vi "One Button Dialog with Timeout.vi"(0 "message":string, 1 "Btn Timeout(-1 s)":i32=-1, 3 "T button name (\"OK\")":string="OK", 5 "Parent Wnd(Caller By Default)":refnum<vi>) -> (7 "true":bool)   [LabVIEW 2017]
doc: "Shows a one-button dialog carrying the message and the button name given, and closes it automatically after Btn Timeout(-1 s) seconds. A negative timeout disables the automatic close."
uses:
  a539abf7-d72e-4e1a-867b-c48a8ed28406.vi
panel:
  out "font":T1
  in  "btn":bool
  out "String":string
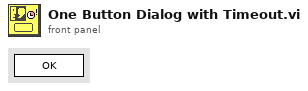
[diagram p1: front panel]
types:
  T1 = cluster{"Font Name:":string, "Size":i16, "Strikeout?":bool, "Italic?":bool, "Underline?":bool, "Outline?":bool, "Shadow?":bool, "Bold?":bool}
  T2 = typedef "LVFontTypeDef.ctl" = cluster{"Font Name":string, "Size":u16, "Bold":bool, "Italic":bool, "Underline":bool, "Strikeout":bool, "Color":u32}
  T3 = cluster{"left":i16, "top":i16, "right":i16, "bottom":i16}
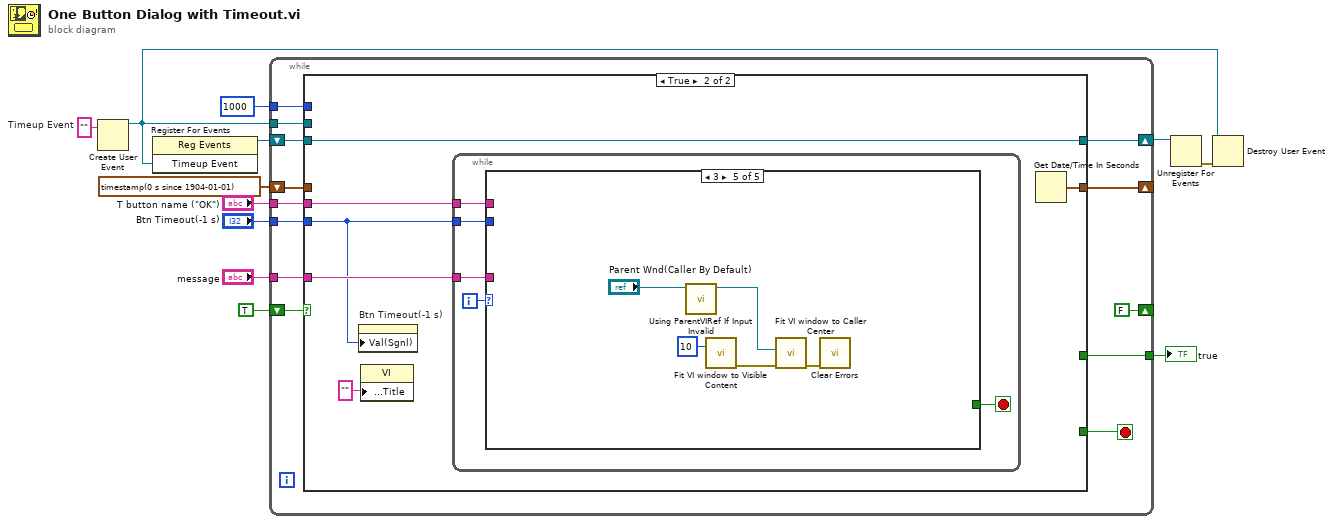
[diagram p0: block diagram]
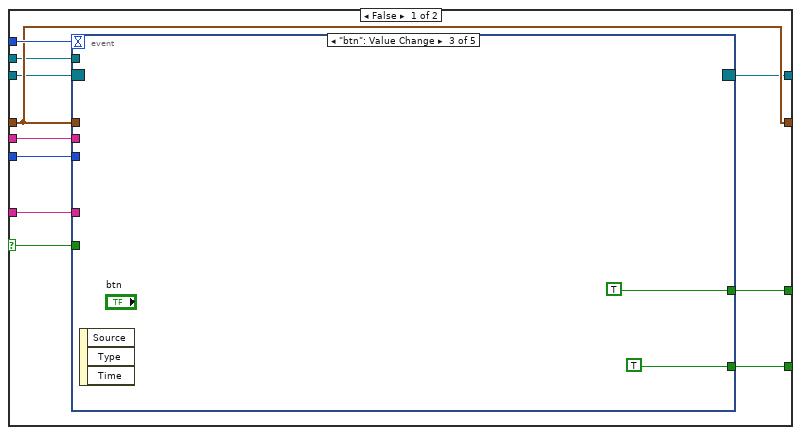
[diagram p2: hidden frame]
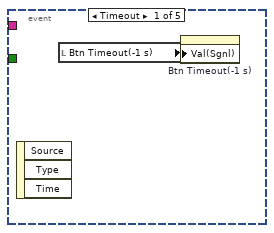
[diagram p3: hidden frame]
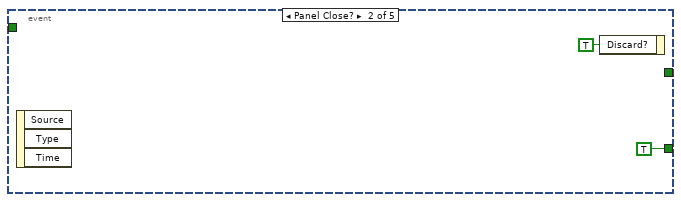
[diagram p4: hidden frame]
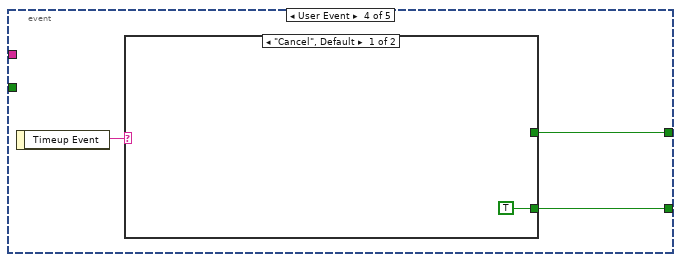
[diagram p5: hidden frame]
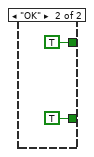
[diagram p6: hidden frame]
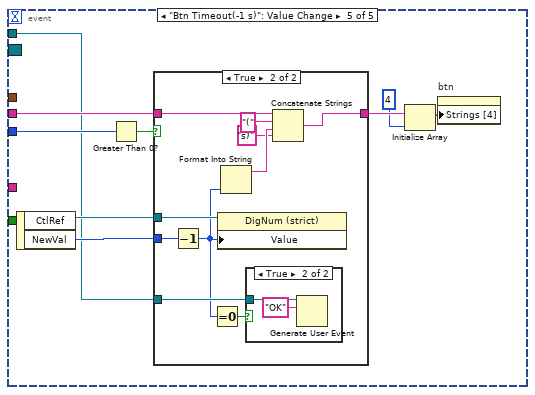
[diagram p7: hidden frame]
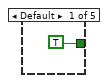
[diagram p10: hidden frame]
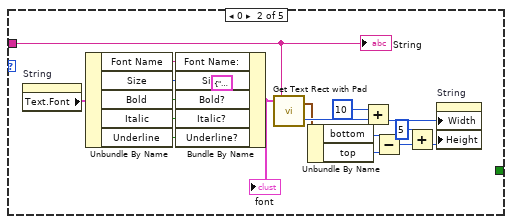
[diagram p11: hidden frame]
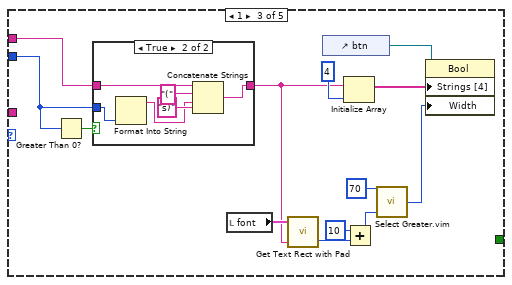
[diagram p12: hidden frame]
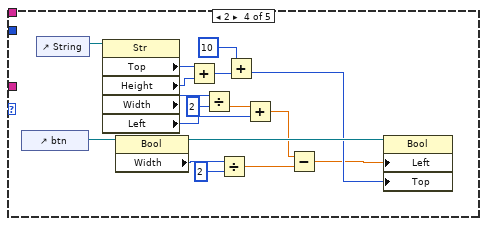
[diagram p14: hidden frame]
diagram:
  w5 = ""  # Timeup Event
  n1 = Create User Event(user event datatype=w5) -> (user event=w1:refnum<user-event>)  [unwired: 1 in, 1 out]
  n2 = register-events(w1) -> (reference out=w4:refnum<event-registration>)  [unwired: 2 in, 1 out]
  n3 = while {
    tunnel: [w24] -> w12
    tunnel: "T button name (\"OK\")" -> [w20]
    tunnel: "message" -> [w21]
    shift-right: [FALSE] -> _
    shift-left: TRUE -> [w23]
    tunnel: "Btn Timeout(-1 s)" -> [w19]
    shift-right: [w18] -> _
    shift-left: timestamp(0 s since 1904-01-01) ("seconds since 1Jan1904") -> [w17]
    tunnel: 1000 -> [w16]
    shift-right: [w14] -> w3
    shift-left: w4 -> [w15]
    tunnel: w1 -> [w13]
    stop <- w25 stop-if-true
    n4 = case shown="True" w23 {
      selector: w23 -> [w33 _]
      tunnel: [w36 _] -> w25
      tunnel: [w35 _] -> w24
      tunnel: w16 -> [w34 _]
      tunnel: w21 -> [w30 w73]
      tunnel: w20 -> [w32 w72]
      tunnel: w19 -> [w31 w71]
      tunnel: [w29 w75] -> w18
      tunnel: w17 -> [w29 _]
      tunnel: w15 -> [w28 w74]
      tunnel: [w27 w74] -> w14
      tunnel: w13 -> [w26 _]
      frame False {
        n5 = event shown="[2] \"btn\": Value Change" {
          selector: w28 -> [_ _ _ _ _]
          dyn-events: [_ _ _ _ _] -> w27
          timeout: w34 -> [_ _ _ _ _]
          tunnel: [_ TRUE ("Discard?") TRUE ("Discard?") w43 _] -> w36
          tunnel: [_ _ TRUE w42 _] -> w35
          tunnel: w33 -> [_ _ _ _ _]
          tunnel: w32 -> [_ _ _ _ w56]
          tunnel: w31 -> [_ _ _ _ w54]
          tunnel: w30 -> [_ _ _ _ _]
          tunnel: w29 -> [_ _ _ _ _]
          tunnel: w26 -> [_ _ _ _ w48]
          event Timeout {
            n6 = event-data() -> ()  [unwired: 1 in, 3 out]
            n7 = local read "Btn Timeout(-1 s)"() -> (w37:i32)
            n8 = property on="Btn Timeout(-1 s)" class="DigNum (strict)"("Val(Sgnl)"=w37) -> ()  [unwired: 2 in, 2 out]
          }
          event Panel Close? {
            n9 = event-data() -> ()  [unwired: 1 in, 3 out]
            n10 = event-data("Discard?"=TRUE) -> ()  [unwired: 1 in, 1 out]
          }
          event "btn": Value Change {
            n11 = event-data() -> ()  [unwired: 1 in, 3 out]
          }
          event User Event {
            n12 = event-data() -> ("Timeup Event"=w44:string)  [unwired: 1 in]
            n13 = case shown="\"Cancel\", Default" w44 {
              tunnel: [TRUE ("Discard?") TRUE ("Discard?")] -> w43
              tunnel: [_ TRUE ("Discard?")] -> w42
              frame "Cancel", Default {
              }
              frame "OK" {
              }
            }
          }
          event "Btn Timeout(-1 s)": Value Change {
            n14 = event-data() -> ("CtlRef"=w50:refnum<vi>, "NewVal"=w49:i32)  [unwired: 1 in]
            n15 = Greater Than 0?(x=w54) -> (x > 0?=w55:bool)
            n16 = case shown="True" w55 {
              tunnel: w56 -> [w57 w67]
              tunnel: [w57 w63] -> w53
              tunnel: w49 -> [_ w62]
              tunnel: w50 -> [_ w61]
              tunnel: w48 -> [_ w59]
              frame False {
              }
              frame True {
                n17 = Decrement(x=w62) -> (x-1=w58:i32)
                n18 = Equal To 0?(x=w58) -> (x = 0?=w60:bool)
                n19 = property class="DigNum (strict)"(reference=w61, "Value"=w58) -> ()  [unwired: 1 in, 2 out]
                n20 = Format Into String(w58) -> (resulting string=w66:string)  [unwired: 3 in, 1 out]
                n21 = case shown="True" w60 {
                  tunnel: w59 -> [_ w69]
                  frame False {
                  }
                  frame True {
                    n22 = Generate User Event(user event=w69, event data cluster="OK" ("event data")) -> ()  [unwired: 2 in, 2 out]
                  }
                }
                n23 = Concatenate Strings(w67, "(" ("string"), w66, "s)" ("string")) -> (w63:string)
              }
            }
            n24 = Initialize Array(w53, 4 ("dimension size")) -> (w52:string[])
            n25 = property on="btn" class="Bool"("Strings [4]"=w52) -> ()  [unwired: 2 in, 2 out]
          }
        }
      }
      frame True {
        n26 = property on="Btn Timeout(-1 s)" class="DigNum (strict)"("Val(Sgnl)"=w71) -> ()  [unwired: 2 in, 2 out]
        n27 = property class="VI"("Front Panel.Title"="" ("Front Panel Window:Title")) -> ()  [unwired: 2 in, 2 out]
        n28 = while {
          tunnel: w73 -> [w80]
          tunnel: w72 -> [w77]
          tunnel: w71 -> [w76]
          i -> [w79]
          stop <- w78 stop-if-true
          n29 = case shown="3" w79 {
            tunnel: w80 -> [_ w98 _ _ _]
            tunnel: [TRUE _ _ _ _] -> w78
            tunnel: w77 -> [_ _ w109 _ _]
            tunnel: w76 -> [_ _ w108 _ _]
            frame Default {
            }
            frame 0 {
              n30 = property on="String" class="Str"() -> ("Text.Font"=w99:T2)  [unwired: 2 in, 2 out]
              n31 = Unbundle By Name(w99) -> ("Font Name"=w95:string, "Size"=w94:u16, "Bold"=w93:bool, "Italic"=w91:bool, "Underline"=w92:bool)
              n32 = Bundle By Name(cluster=T1 {"Font Name:"="", "Size"=0, "Strikeout?"=FALSE, "Italic?"=FALSE, "Underline?"=FALSE, "Outline?"=FALSE, "Shadow?"=FALSE, "Bold?"=FALSE} ("Font"), "Font Name:"=w95, "Size"=w94, "Bold?"=w93, "Italic?"=w91, "Underline?"=w92) -> (w96:T1)
              "font" <- w96
              n33 = call "Get Text Rect with Pad.vi"("Text"=w98, "Font"=w96) -> ("Width"=w90:i16, "Rect"=w89:T3)  [unwired: 1 in]
              n34 = Unbundle By Name(w89) -> ("bottom"=w86:i16, "top"=w88:i16)
              n35 = Add(x=i16 10, y=w90) -> (x+y=w83:i16)
              n36 = Subtract(x=w86, y=w88) -> (x-y=w87:i16)
              n37 = Add(x=i16 5, y=w87) -> (x+y=w85:i16)
              n38 = property on="String" class="Str"("Width"=w83, "Height"=w85) -> ()  [unwired: 2 in, 2 out]
              "String" <- w98
            }
            frame 1 {
              n39 = Greater Than 0?(x=w108) -> (x > 0?=w112:bool)
              n40 = case shown="True" w112 {
                tunnel: w109 -> [w113 w119]
                tunnel: [w113 w116] -> w105
                tunnel: w108 -> [_ w114]
                frame False {
                }
                frame True {
                  n41 = Format Into String(w114) -> (resulting string=w115:string)  [unwired: 3 in, 1 out]
                  n42 = Concatenate Strings(w119, "(" ("string"), w115, "s)" ("string")) -> (w116:string)
                }
              }
              n43 = local read "font"() -> (w106:T1)
              n44 = call "Get Text Rect with Pad.vi"("Text"=w105, "Font"=w106) -> ("Width"=w104:i16)  [unwired: 1 in, 1 out]
              n45 = control-ref of="btn"() -> (w107:refnum<vi>)
              n46 = Initialize Array(w105, 4 ("dimension size")) -> (w111:string[])
              n47 = Add(x=i16 10, y=w104) -> (x+y=w101:i16)
              n48 = call "Select Greater.vim"("A"=70, "B"=w101) -> ("lesser"=w100:i32)  [unwired: 3 in]
              n49 = property on="Property Node" class="Bool"(reference=w107, "Strings [4]"=w111, "Width"=w100) -> ()  [unwired: 1 in, 2 out]
            }
            frame 2 {
              n50 = control-ref of="btn"() -> (w131:refnum<vi>)
              n51 = control-ref of="String"() -> (w136:refnum<vi>)
              n52 = property class="Str"(reference=w136) -> ("Top"=w135:i32, "Height"=w134:u32, "Width"=w126:u32, "Left"=w132:i32)  [unwired: 1 in, 2 out]
              n53 = property class="Bool"(reference=w131) -> (reference out=w130:refnum<vi>, "Width"=w124:u32)  [unwired: 1 in, 1 out]
              n54 = Add(x=w135, y=w134) -> (x+y=w133:u32)
              n55 = Divide(x=w126, y=u32 2) -> (x/y=w127:dbl)
              n56 = Divide(x=w124, y=u32 2) -> (x/y=w121:dbl)
              n57 = Add(x=u32 10, y=w133) -> (x+y=w129:u32)
              n58 = Add(x=w127, y=w132) -> (x+y=w122:dbl)
              n59 = Subtract(x=w122, y=w121) -> (x-y=w120:dbl)
              n60 = property class="Bool"(reference=w130, "Left"=w120, "Top"=w129) -> ()  [unwired: 1 in, 2 out]
            }
            frame 3 {
              n61 = call "Using ParentVIRef If Input Invalid.vi"("VI Ref (calling VI)"="Parent Wnd(Caller By Default)") -> ("VI Ref"=w137:refnum<vi>)  [unwired: 5 in, 1 out]
              n62 = call "Fit VI window to Visible Content.vi"("border spacing (2 px)"=10) -> ("error out"=w141:errorcluster)  [unwired: 5 in, 1 out]
              n63 = call "Fit VI window to Caller Center.vi"("Error In"=w141, "Background VI Ref (Callee's Caller)"=w137) -> ("Error Out"=w140:errorcluster)  [unwired: 4 in, 1 out]
              n64 = call <vilib>:"Clear Errors.vi"("error in (no error)"=w140) -> ()  [unwired: 5 in, 2 out]
            }
          }
        }
        n65 = Get Date/Time In Seconds() -> (seconds since 1Jan1904=w75:timestamp)
      }
    }
  }
  "true" <- w12
  n66 = Unregister For Events(event registration refnum=w3) -> (error out=w2:errorcluster)  [unwired: 1 in]
  n67 = Destroy User Event(user event=w1, error in=w2) -> ()  [unwired: 1 out]
